vi "Wait.Gui.Update.vi"(8 "error in (no error)":errorcluster, 10 "Status":string) -> (0 "error out":errorcluster)   [LabVIEW 2015]
uses:
  Wait.Gui.Action.ctl
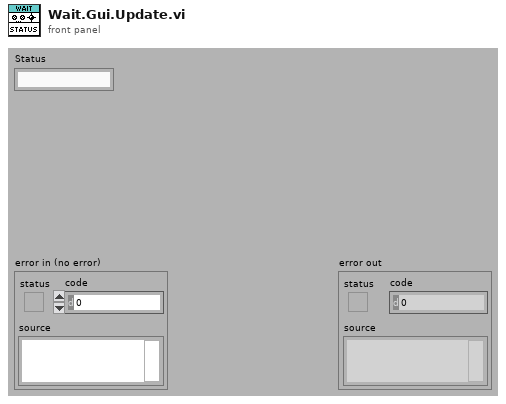
[diagram p1: front panel]
types:
  T1 = typedef "Wait.Gui.Action.ctl" = enum32{"idle", "constructor", "destructor", "--- GuiServerWait ---", "open FP", "close FP", "update status", "update msg", "update progbar"}
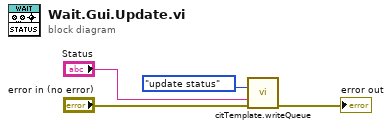
[diagram p0: block diagram]
diagram:
  n1 = call "citTemplate.writeQueue.vi"("event in (if not connected:all statemachine with data event)"=Wait.Gui.Action."update status" ("Action"), "data in"="Status", "error in (no error)"="error in (no error)") -> ("error out"=→"error out":errorcluster)  [unwired: 12 in]
